vi "Take_scan.vi"(7 "batch_shg location (should be on Desktop)":path, 8 "Output File name":string, 9 "Number of Accumulations":i32, 10 "Exposure Time (s)":dbl format="%#_13g", 11 "SHG_scat_scan.exe location":path) -> ()   [LabVIEW 2017]
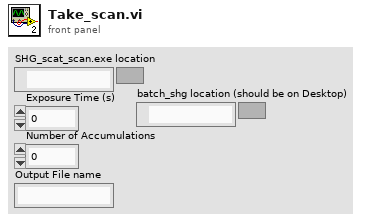
[diagram p1: front panel]
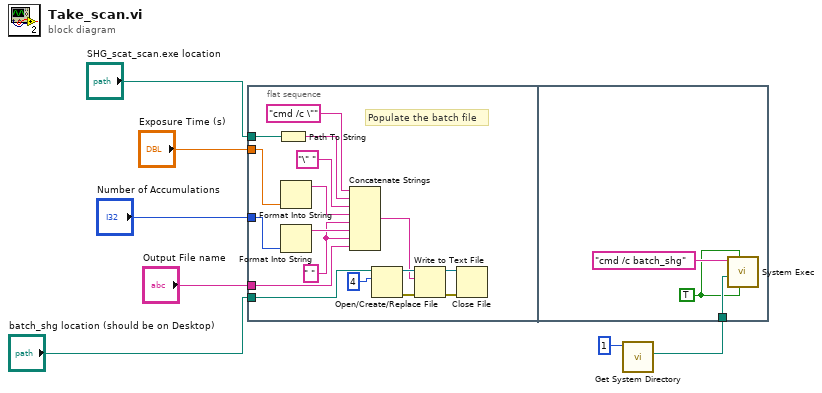
[diagram p0: block diagram]
diagram:
  n1 = flat-sequence {
    tunnel: "Exposure Time (s)" -> [w14]
    tunnel: "Number of Accumulations" -> [w15]
    tunnel: "batch_shg location (should be on Desktop)" -> [w24]
    tunnel: "SHG_scat_scan.exe location" -> [w18]
    tunnel: "Output File name" -> [w9]
    tunnel: w2 -> [w26]
    frame #0 {
      w10 = " "
      # "Populate the batch file"
      n2 = Path To String(path=w18) -> (string=w17:string)
      n3 = Format Into String(w14) -> (resulting string=w13:string)  [unwired: 3 in, 1 out]
      n4 = Format Into String(w15) -> (resulting string=w12:string)  [unwired: 3 in, 1 out]
      n5 = Concatenate Strings("cmd /c \"", w17, "\" ", w13, w10, w12, w10, w9) -> (w11:string)
      n6 = Open/Create/Replace File(file path (use dialog)=w24, operation (0:open)=4) -> (refnum out=w23:refnum<file>, error out=w22:errorcluster)  [unwired: 4 in, 1 out]
      n7 = Write to Text File(file (use dialog)=w23, text=w11, error in=w22) -> (refnum out=w20:refnum<file>, error out=w21:errorcluster)  [unwired: 1 in, 1 out]
      n8 = Close File(refnum=w20, error in=w21) -> ()  [unwired: 2 out]
    }
    frame #1 {
      w25 = TRUE
      n9 = call <vilib>:"System Exec.vi"("run minimized? (F)"=w25, "wait until completion? (T)"=w25, "working directory"=w26, "command line"="cmd /c batch_shg") -> ()  [unwired: 4 in, 4 out]
    }
  }
  n10 = call <vilib>:"Get System Directory.vi"("system directory type"=1) -> ("system directory"=w2:path)  [unwired: 10 in]
